vi "Fix Bad Page.vi"(10 "Page":i32[](array[numeric]), 11 "Rules":i32[][](array[numeric])) -> (2 "Fixed Page":i32[](array[numeric]))   [LabVIEW 2024]
panel:
  out "Page 2":i32[](array[numeric])
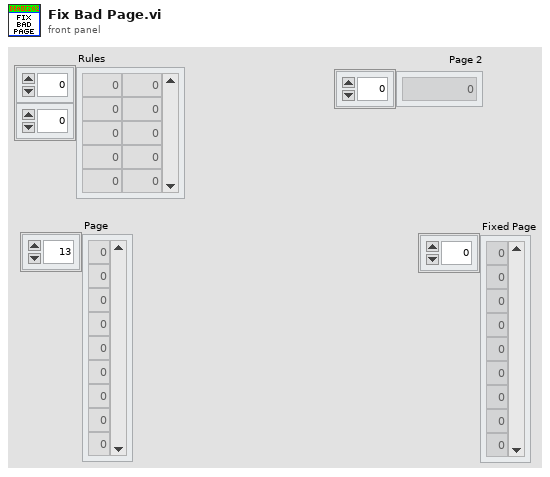
[diagram p1: front panel]
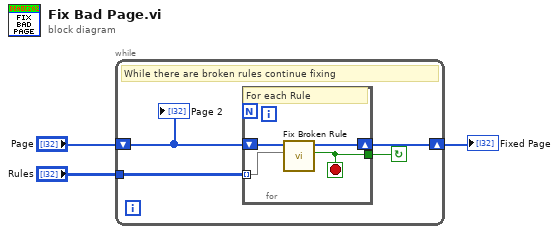
[diagram p0: block diagram]
diagram:
  n1 = while {
    tunnel: "Rules" -> [w7]
    shift-right: [w5] -> w1
    shift-left: "Page" -> [w6]
    stop <- w4 continue-if-true
    # "While there are broken rules continue fixing"
    n2 = for {
      tunnel: w7 -> [w11] mode=indexing
      tunnel: [w9] -> w4
      shift-right: [w8] -> w5
      shift-left: w6 -> [w10]
      stop <- w9 stop-if-true
      # "For each Rule"
      n3 = call "Fix Broken Rule.vi"("Rule"=w11, "Page"=w10) -> ("Fixed Out"=w9:bool, "Page Out"=w8:i32[])  [unwired: 8 in]
    }
    "Page 2" <- w6
  }
  "Fixed Page" <- w1
